vi "SSCP_readSocket.vi"(3 "error in":errorcluster, 5 "connection in":refnum<k5>) -> (0 "error out":errorcluster, 1 "payload":string, 2 "connection out":refnum<k5>)   [LabVIEW 2020]
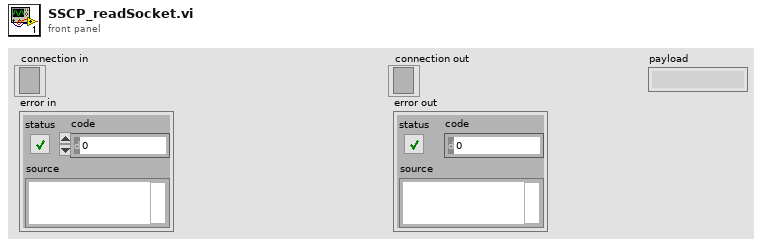
[diagram p1: front panel]
types:
  T1 = enum16{"Standard", "Buffered", "CRLF", "Immediate"}
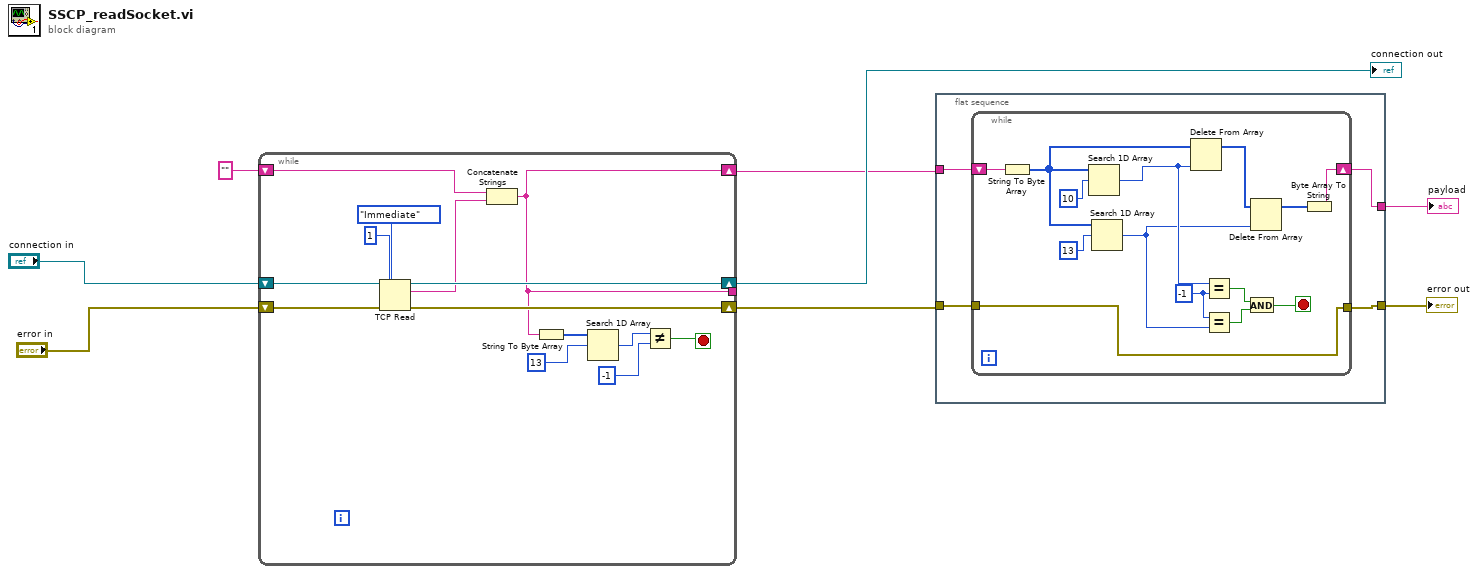
[diagram p0: block diagram]
diagram:
  n1 = while {
    tunnel: [w9] -> _
    shift-right: [w18] -> w3
    shift-left: "error in" -> [w22]
    shift-right: [w17] -> w6
    shift-left: "connection in" -> [w21]
    shift-right: [w9] -> w4
    shift-left: "" -> [w16]
    stop <- w10 stop-if-true
    n2 = TCP Read(connection ID=w21, bytes to read=1, error in (no error)=w22, 7:T1."Immediate" ("mode (standard)")) -> (connection ID out=w17:refnum<k5>, data out=w15:string, error out=w18:errorcluster)  [unwired: 1 in]
    n3 = Concatenate Strings(w16, w15) -> (w9:string)
    n4 = String To Byte Array(string=w9) -> (unsigned byte array=w14:u8[])
    n5 = Search 1D Array(1D array=w14, element=u8 13) -> (index of element=w12:i32)  [unwired: 1 in]
    n6 = Not Equal?(x=w12, y=-1) -> (x != y?=w10:bool)
  }
  "connection out" <- w6
  n7 = flat-sequence {
    tunnel: w4 -> [w26]
    tunnel: w3 -> [w24]
    tunnel: [w23] -> w2
    tunnel: [w25] -> w1
    frame #0 {
      n8 = while {
        tunnel: w24 -> [w27]
        shift-right: [w34] -> w25
        shift-left: w26 -> [w40]
        tunnel: [w27] -> w23
        stop <- w28 stop-if-true
        w31 = -1 ("y")
        n9 = String To Byte Array(string=w40) -> (unsigned byte array=w37:u8[])
        n10 = Search 1D Array(1D array=w37, element=u8 10) -> (index of element=w33:i32)  [unwired: 1 in]
        n11 = Search 1D Array(1D array=w37, element=u8 13) -> (index of element=w32:i32)  [unwired: 1 in]
        n12 = Delete From Array(array=w37, index=w33) -> (array with subset deleted=w36:u8[])  [unwired: 1 in, 1 out]
        n13 = Equal?(x=w33, y=w31) -> (x = y?=w30:bool)
        n14 = Equal?(x=w31, y=w32) -> (x = y?=w29:bool)
        n15 = And(x=w30, y=w29) -> (x .and. y?=w28:bool)
        n16 = Delete From Array(array=w36, index=w32) -> (array with subset deleted=w35:u8[])  [unwired: 1 in, 1 out]
        n17 = Byte Array To String(unsigned byte array=w35) -> (string=w34:string)
      }
    }
  }
  "error out" <- w2
  "payload" <- w1
